vi "Create List Of FPGA in this Schedule.vi"(8 "error in (no error)":errorcluster, 11 "Schedule in":refnum<class "Schedule.lvclass">) -> (0 "error out":errorcluster, 3 "Schedule out":refnum<class "Schedule.lvclass">)   [LabVIEW 2020, in "CIRCUS_uServices.lvlib" / "Run Utilities.lvlib" / "Schedule.lvclass"]
doc: "Go over the entire schedule and create a list of Kaslis that are used in the Schedule"
uses:
  Schedule.lvclass
  Schedule.lvclass/Schedule.ctl
  Cell/Schedule Cell.lvclass
  b09dac26-fe60-4391-a7a8-81447650faa1.vi
  9bc96d9d-9184-4bd2-95c3-fe24546c86f6.vi
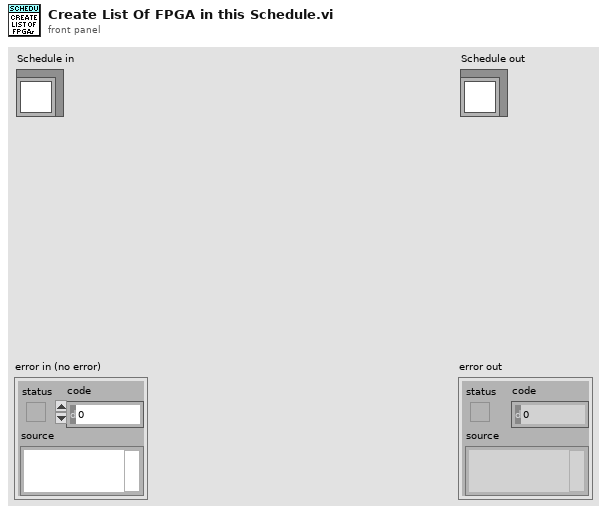
[diagram p1: front panel]
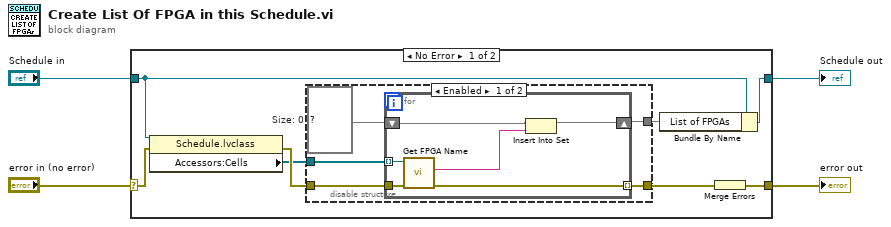
[diagram p0: block diagram]
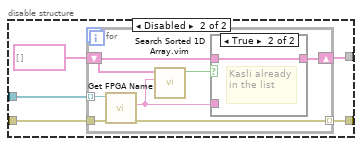
[diagram p2: hidden frame]
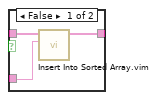
[diagram p3: hidden frame]
diagram:
  n1 = case shown="No Error" "error in (no error)" {
    selector: "error in (no error)" -> [w12 w41]
    tunnel: [w6 w41] -> w3
    tunnel: [w8 w40] -> w1
    tunnel: "Schedule in" -> [w9 w40]
    frame No Error {
      n2 = property class="Schedule.lvclass"(reference=w9, error in=w12) -> (error out=w11:errorcluster, "Accessors:Cells"=w10:refnum<class "Schedule Cell.lvclass">[])  [unwired: 1 out]
      n3 = disable-structure shown="Enabled" {
        disable-tunnel: w11 -> [w17 w28]
        disable-tunnel: w10 -> [w16 w27]
        disable-tunnel: [w15 w26] -> w7
        disable-tunnel: [w14 w24] -> w5
        frame Enabled {
          w13 = set{string} {}  # Size: 0
          n4 = for {
            tunnel: w16 -> [w22] mode=indexing
            tunnel: w17 -> [w23]
            shift-right: [w19] -> w14
            shift-left: w13 -> [w20]
            tunnel: [w21] -> w15 mode=indexing
            n5 = call-dynamic "Get FPGA Name.vi"("error in (no error)"=w23, "Schedule Cell in"=w22) -> ("error out"=w21:errorcluster, "FPGA Name"=w18:string)  [unwired: 7 in, 1 out]
            n6 = Insert Into Set(10:w18, 11:w20) -> (3:w19:set{string})  [unwired: 1 out]
          }
        }
        frame Disabled {
          n7 = for {
            tunnel: w27 -> [w34] mode=indexing
            tunnel: w28 -> [w35]
            shift-right: [w32] -> w24
            shift-left: string[] [] -> [w31]
            tunnel: [w33] -> w26 mode=indexing
            n8 = call-dynamic "Get FPGA Name.vi"("error in (no error)"=w35, "Schedule Cell in"=w34) -> ("error out"=w33:errorcluster, "FPGA Name"=w30:string)  [unwired: 7 in, 1 out]
            n9 = call "Search Sorted 1D Array.vim"("element"=w30, "sorted 1D array"=w31) -> ("found?"=w29:bool)  [unwired: 8 in, 1 out]
            n10 = case shown="True" w29 {
              tunnel: [w38 w39] -> w32
              tunnel: w31 -> [w37 w39]
              tunnel: w30 -> [w36 _]
              frame False {
                n11 = call "Insert Into Sorted Array.vim"("element"=w36, "sorted array in"=w37) -> ("sorted array out"=w38:string[])  [unwired: 9 in]
              }
              frame True {
                # "Kasli already in the list"
              }
            }
          }
        }
      }
      n12 = Bundle By Name(cluster=w9, "List of FPGAs"=w5) -> (w8:refnum<class "Schedule.lvclass">)
      n13 = Merge Errors(w7) -> (w6:errorcluster)
    }
    frame Error {
    }
  }
  "error out" <- w3
  "Schedule out" <- w1
